vi "Is Child Path -- JKI State Machine Editor.vi"(1 "Path":path, 2 "Parent Directory":path) -> (0 "is Child Path?":bool)   [LabVIEW 2013]
uses:
  <userlib>/_OpenG.lib/file/file.llb/Compare Two Paths - Scalar__ogtk.vi
panel:
  # "Copyright © 2008 JKI. All rights reserved.\n\nAuthor: Jim Kring [jim.kring@jameskring.com]\n\nThis library is provided \"AS IS\" ,WITHOUT WARRANTIES OR \nCONDITIONS OF ANY KIND, either express or implied.\n\nJKI -- http://www.jameskring.com"
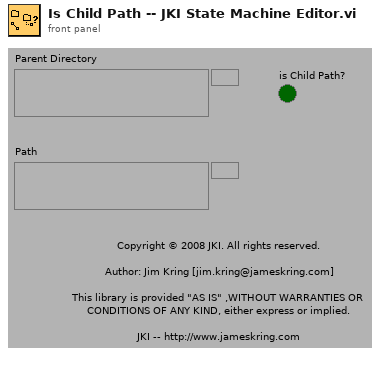
[diagram p1: front panel]
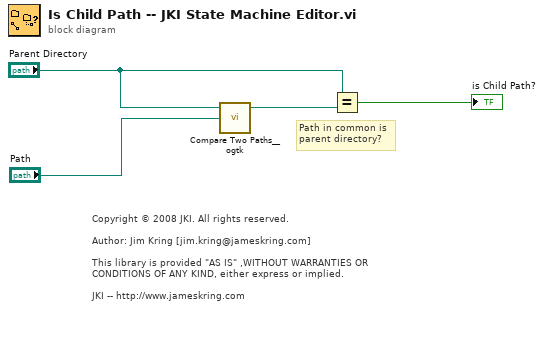
[diagram p0: block diagram]
diagram:
  # "Copyright © 2008 JKI. All rights reserved.\n\nAuthor: Jim Kring [jim.kring@jameskring.com]\n\nThis library is provided \"AS IS\" ,WITHOUT WARRANTIES OR \nCONDITIONS OF ANY KIND, either express or implied.\n\nJKI -- http://www.jameskring.com"
  # "Path in common is parent directory?"
  n1 = call-poly <userlib>:"Compare Two Paths__ogtk.vi"("path2"="Path", "path1"="Parent Directory") -> ("common path"=w2:path)  [unwired: 1 in, 2 out]
  n2 = Equal?(x="Parent Directory", y=w2) -> (x = y?=→"is Child Path?":bool)
